vi "Read Limits.vi"(8 "error in (no error)":errorcluster, 11 "Alarms in":refnum<class "HK Alarms.lvclass">) -> (0 "error out":errorcluster, 2 "Limits":T1, 3 "Alarms out":refnum<class "HK Alarms.lvclass">)   [LabVIEW 2019, in "HK Alarms.lvclass"]
uses:
  HK Alarms/HK Alarms.lvclass
  HK Item/HK Channel Settings Limits.ctl
  HK Alarms/HK Alarms.lvclass/HK Alarms.ctl
  HK Item/HK Item.lvclass
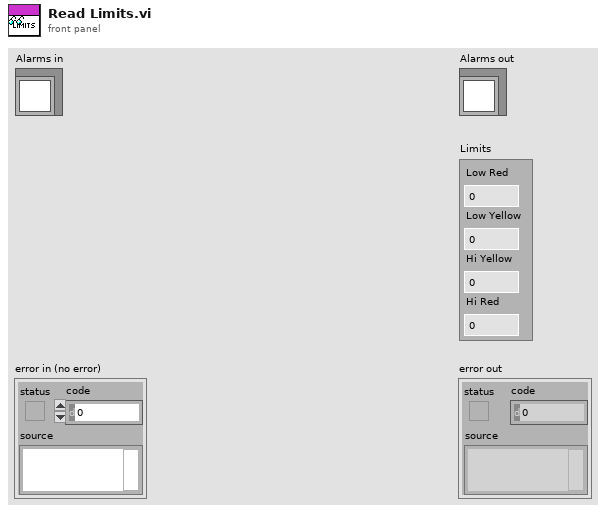
[diagram p1: front panel]
types:
  T1 = typedef "HK Item.lvclass/HK Channel Settings Limits.ctl" = cluster{"Low Red":dbl, "Low Yellow":dbl, "Hi Yellow":dbl, "Hi Red":dbl}
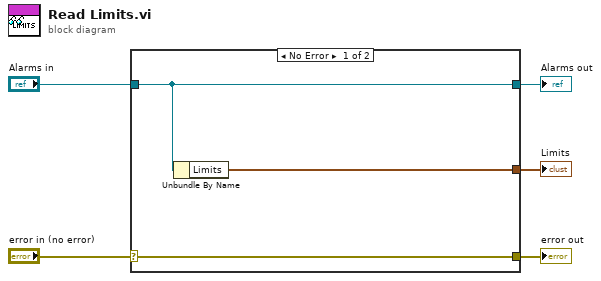
[diagram p0: block diagram]
diagram:
  n1 = case shown="No Error" "error in (no error)" {
    selector: "error in (no error)" -> [w8 w9]
    tunnel: [w8 w9] -> w4
    tunnel: [w7 w10] -> w2
    tunnel: "Alarms in" -> [w7 w10]
    tunnel: [w6 _] -> w1
    frame No Error {
      n2 = Unbundle By Name(w7) -> ("Limits"=w6:T1)
    }
    frame Error {
    }
  }
  "error out" <- w4
  "Alarms out" <- w2
  "Limits" <- w1
